vi "Get System Info.vi"() -> ()   [LabVIEW 2015, in "SMI.lvlib"]
uses:
  classes/Controller/Controls/NetworkDevice.ctl
  classes/Controller/Controls/DeviceInformation.ctl
  classes/Controller/Controls/NetworkAdapterSettings.ctl
  classes/Chassis/Controls/ChassisInformation.ctl
  classes/Module/Controls/ModuleInformation.ctl
  SMI.lvlib
  classes/SysCfg Device/SysCfg Device.lvclass
  classes/Controller/Controller.lvclass
  classes/Chassis/Chassis.lvclass
  classes/Module/Module.lvclass
panel:
  out "Chassis Information":T3 {"Remote Chassis"."Modules"."Module Code" format="%.0x"; "Local Chassis"."Modules"."Module Code" format="%.0x"; "Local Chassis"."Chassis"."Product ID" format="%.0x"}
  out "error out":errorcluster
  out "Controller Information":T4={"System Hardware Reference"=refnum, "Vendor Name"="", "Product Name"="", "Product ID"=0, "Serial Number"="", "Device Information"={"Resource"="", "Device Class"="", "System Start Time"=timestamp(0 s since 1904-01-01), "Current Time"=timestamp(0 s since 1904-01-01), "Time Zone"="", "Firmware Revision"="", "Image Title"="", "Image Version"="", "System Status"="", "Credential type"=enum."None/Unlocked", "User Added"=FALSE}, "Primary Network Adapter"={"IP Address"="", "MAC Address"="", "IP Address Request Mode"=1, "SubnetMask"="", "Gateway"="", "DNS Server"="", "Adapter Mode"=1, "Adapter Type"=1}, "Secondary Network Adapters"=[]} {"Product ID" format="%.0x"; "Primary Network Adapter"."IP Address Request Mode" items=["Static"=1, "DHCP/Link Local"=2, "Link-Local Only"=4, "DHCP Only"=8]; "Primary Network Adapter"."Adapter Type" items=["Ethernet"=1, "WLAN"=2]; "Primary Network Adapter"."Adapter Mode" items=["Disabled"=1, "TCP/IP Ethernet"=2, "Deterministic"=4, "EtherCAT"=8, "TCP/IP WLAN Connect"=32, "TCP/IP WLAN Create"=64]; "Secondary Network Adapters"."IP Address Request Mode" items=["Static"=1, "DHCP/Link Local"=2, "Link-Local Only"=4, "DHCP Only"=8]; "Secondary Network Adapters"."Adapter Type" items=["Disabled"=1, "TCP/IP Ethernet"=2, "Deterministic"=4, "EtherCAT"=8, "TCP/IP WLAN Connect"=32, "TCP/IP WLAN Create"=64]; "Secondary Network Adapters"."Adapter Mode" items=["Disabled"=1, "TCP/IP Ethernet"=2, "Deterministic"=4, "EtherCAT"=8, "TCP/IP WLAN Connect"=32, "TCP/IP WLAN Create"=64]}
  in  "NI Auth":cluster{"User Name":string, "Password":string}[](array[cluster])
  in  "Target Address":string
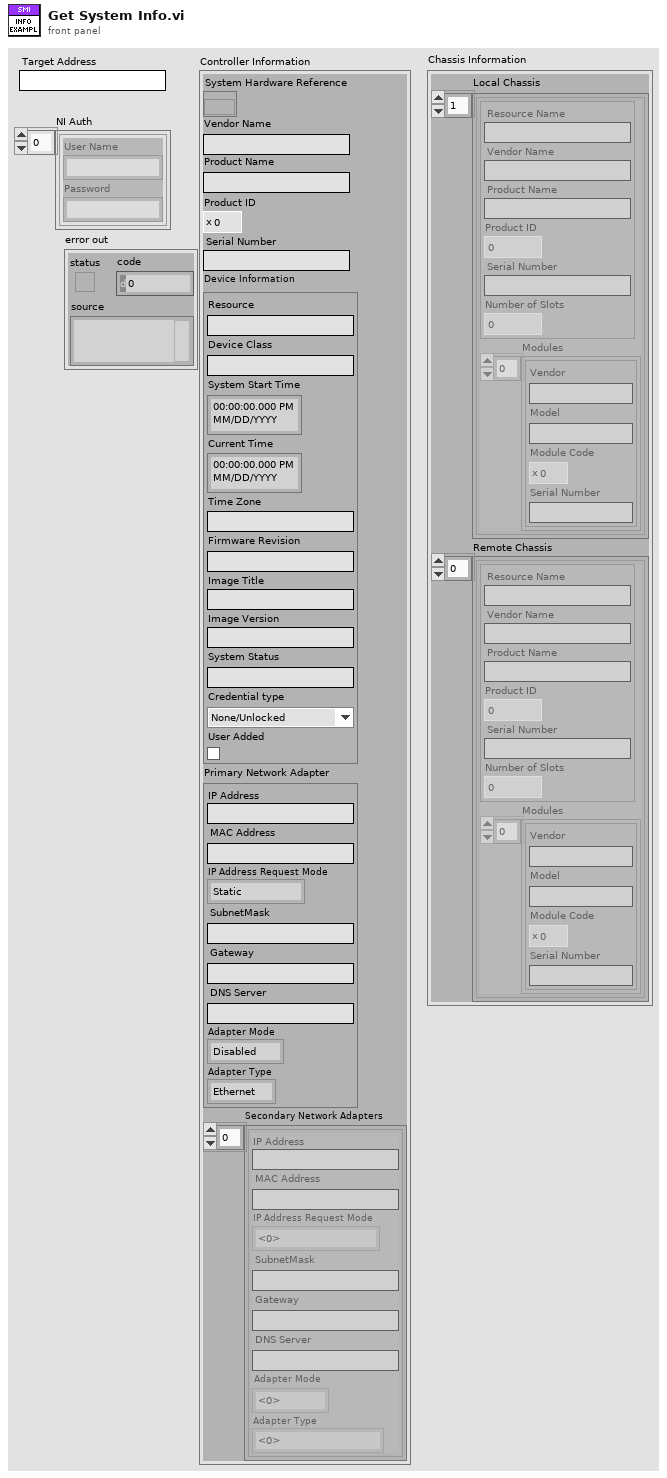
[diagram p1: front panel]
types:
  T1 = typedef "SMI.lvlib/Chassis.lvclass/ChassisInformation.ctl" = cluster{"Resource Name":string, "Vendor Name":string, "Product Name":string, "Product ID":u32, "Serial Number":string, "Number of Slots":i32}
  T2 = typedef "SMI.lvlib/Module.lvclass/ModuleInformation.ctl" = cluster{"Vendor":string, "Model":string, "Module Code":u32, "Serial Number":string}
  T3 = cluster{"Local Chassis":cluster{"Chassis":T1, "Modules":T2[]}[], "Remote Chassis":cluster{"Chassis":T1, "Modules":T2[]}[]}
  T4 = typedef "SMI.lvlib/Controller.lvclass/NetworkDevice.ctl" = cluster{"System Hardware Reference":refnum<k20>, "Vendor Name":string, "Product Name":string, "Product ID":u32, "Serial Number":string, "Device Information":T5, "Primary Network Adapter":T6, "Secondary Network Adapters":T6[]}
  T5 = typedef "SMI.lvlib/Controller.lvclass/DeviceInformation.ctl" = cluster{"Resource":string, "Device Class":string, "System Start Time":timestamp, "Current Time":timestamp, "Time Zone":string, "Firmware Revision":string, "Image Title":string, "Image Version":string, "System Status":string, "Credential type":enum16{"None/Unlocked", "FTP Password", "NIAuth Credentials"}, "User Added":bool}
  T6 = typedef "SMI.lvlib/Controller.lvclass/NetworkAdapterSettings.ctl" = cluster{"IP Address":string, "MAC Address":string, "IP Address Request Mode":u32, "SubnetMask":string, "Gateway":string, "DNS Server":string, "Adapter Mode":u32, "Adapter Type":u32}
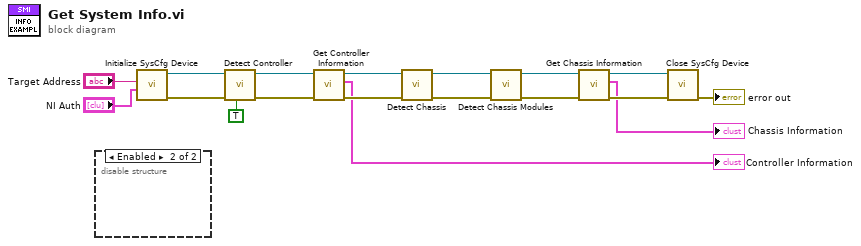
[diagram p0: block diagram]
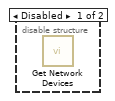
[diagram p2: hidden frame]
diagram:
  n1 = disable-structure shown="Enabled" {
    frame Disabled {
      n2 = call "Get Network Devices.vi"() -> ()  [unwired: 8 in, 4 out]
    }
    frame Enabled {
    }
  }
  n3 = call "Initialize SysCfg Device.vi"("NI Auth"="NI Auth", "Target Address"="Target Address") -> ("error out"=w15:errorcluster, "Controller out"=w16:refnum<class "Controller.lvclass">)  [unwired: 8 in]
  n4 = call "Detect Controller.vi"("Network Adapters"=TRUE, "error in"=w15, "Controller in"=w16) -> ("error out"=w10:errorcluster, "Controller out"=w8:refnum<class "Controller.lvclass">)  [unwired: 7 in]
  n5 = call "Get Controller Information.vi"("error in"=w10, "Controller in"=w8) -> ("error out"=w9:errorcluster, "Device Information"=→"Controller Information":T4, "Controller out"=w7:refnum<class "Controller.lvclass">)  [unwired: 7 in]
  n6 = call "Detect Chassis.vi"("error in"=w9, "Controller in"=w7) -> ("error out"=w6:errorcluster, "Controller out"=w5:refnum<class "Controller.lvclass">)  [unwired: 8 in]
  n7 = call "Detect Chassis Modules.vi"("error in"=w6, "Controller in"=w5) -> ("error out"=w11:errorcluster, "Controller out"=w13:refnum<class "Controller.lvclass">)  [unwired: 8 in]
  n8 = call "Get Chassis Information.vi"("error in"=w11, "Controller in"=w13) -> ("error out"=w4:errorcluster, "Chassis Information"=→"Chassis Information":T3, "Controller out"=w3:refnum<class "Controller.lvclass">)  [unwired: 7 in]
  n9 = call "Close SysCfg Device.vi"("error in"=w4, "Controller in"=w3) -> ("error out"=→"error out":errorcluster)  [unwired: 9 in]
